vi "select_pose_waveforms.vi"(5 "Trace timestamp":timestamp, 6 "Decimated trace":sgl[][][](array[numeric]), 7 "Decimated dt":dbl, 9 "Reference":sgl[][](array[numeric]), 10 "Pose selectors":T2[](array[typedef]), 11 "Waveforms in":waveform(sgl)[](array[waveform])) -> (3 "Waveforms out":waveform(sgl)[](array[waveform]))   [LabVIEW 2013]
uses:
  pose_selector.ctl
  pose_source.ctl
  pose_relative_to.ctl
panel:
  out "Nother dummy":enum16{"At tip", "At RCM", "At KC", "At origin"}(ring)
  in  "Dummy for names":T1
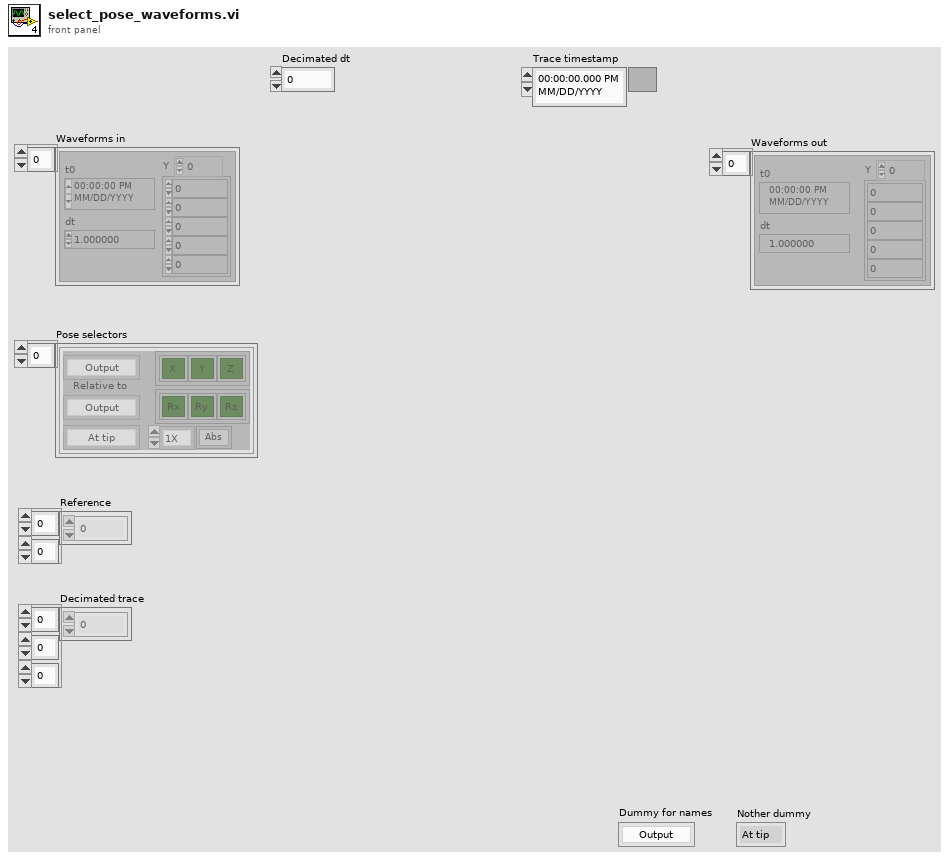
[diagram p1: front panel]
types:
  T1 = typedef "pose_relative_to.ctl" = enum16{"Output", "Handle", "Handle KF", "Goal", "Absolute", "Trace start"}
  T2 = typedef "pose_selector.ctl" = cluster{"Scale":enum16{"1X", "10X", "100X", "1KX", "10KX"}, "Source":T3, "XYZ selector":cluster{"Boolean":bool, "Boolean 2":bool, "Boolean 3":bool}, "RPY selector":cluster{"Boolean":bool, "Boolean 2":bool, "Boolean 3":bool}, "Relative to":T1, "Relative":bool, "Translate":enum16{"At tip", "At RCM", "At KC", "At origin"}}
  T3 = typedef "pose_source.ctl" = enum16{"Output", "Handle", "Handle KF", "Goal", "Absolute"}
  T4 = cluster{"Boolean":bool, "Boolean 2":bool, "Boolean 3":bool}
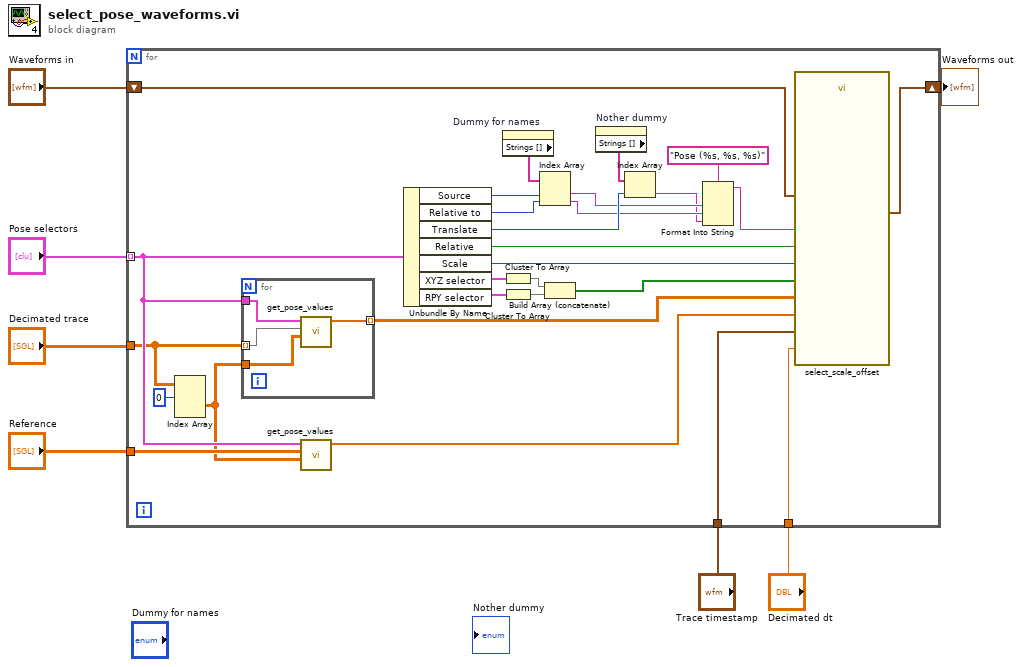
[diagram p0: block diagram]
diagram:
  n1 = for {
    shift-right: [w27] -> w3
    shift-left: "Waveforms in" -> [w28]
    tunnel: "Pose selectors" -> [w23] mode=indexing
    tunnel: "Decimated trace" -> [w10]
    tunnel: "Reference" -> [w24]
    tunnel: "Decimated dt" -> [w26]
    tunnel: "Trace timestamp" -> [w11]
    n2 = Index Array(array=w10, index (dim 0)=0 ("index (page)")) -> (element=w8:sgl[][])  [unwired: 2 in]
    n3 = for {
      tunnel: w10 -> [w39] mode=indexing
      tunnel: w23 -> [w38]
      tunnel: [w37] -> w25 mode=indexing
      tunnel: w8 -> [w36]
      n4 = call "get_pose_values.vi"("First record"=w36, "Trace record"=w39, "Selector"=w38) -> ("XYZ Rx Ry Rz"=w37:dbl[])  [unwired: 8 in]
    }
    n5 = call "get_pose_values.vi"("First record"=w8, "Trace record"=w24, "Selector"=w23) -> ("XYZ Rx Ry Rz"=w22:dbl[])  [unwired: 8 in]
    n6 = Unbundle By Name(w23) -> ("Source"=w20:T3, "Relative to"=w19:T1, "Translate"=w17:enum16{"At tip", "At RCM", "At KC", "At origin"}, "Relative"=w34:bool, "Scale"=w35:enum16{"1X", "10X", "100X", "1KX", "10KX"}, "XYZ selector"=w33:T4, "RPY selector"=w32:T4)
    n7 = property on="Dummy for names" class="Enum (strict)"() -> ("Strings []"=w21:string[])  [unwired: 2 in, 2 out]
    n8 = Cluster To Array(cluster=w33) -> (array=w31:bool[])
    n9 = Cluster To Array(cluster=w32) -> (array=w30:bool[])
    n10 = Index Array(array=w21, index #1=w20, index #2=w19) -> (element #1=w15:string, element #2=w14:string)
    n11 = Build Array (concatenate)(w31, w30) -> (w29:bool[])
    n12 = property on="Nother dummy" class="Enum (strict)"() -> ("Strings []"=w18:string[])  [unwired: 2 in, 2 out]
    n13 = Index Array(array=w18, index=w17) -> (element=w13:string)
    n14 = Format Into String(format string="Pose (%s, %s, %s)", w15, w14, w13) -> (resulting string=w12:string)  [unwired: 2 in, 1 out]
    n15 = call "select_scale_offset.vi"("Waveforms in"=w28, "Points"=w25, "Name"=w12, "Selector"=w29, "Scale"=w35, "Relative"=w34, "Decimated dt"=w26, "Trace timestamp"=w11, "Reference"=w22) -> ("Waveforms out"=w27:waveform(sgl)[])  [unwired: 6 in]
  }
  "Waveforms out" <- w3
